vi "Change File True.vi"(0 "error in":errorcluster, 1 "Numeric in":u16, 2 "Ring":refnum<vi>) -> (7 "error out":errorcluster, 8 "Numeric out":u16, 9 "Change song?":bool)   [LabVIEW 2019]
doc: "Checks if the Ring has been changed or if the application has finished reading the audio file and sends a boolean value depending the condition was true."
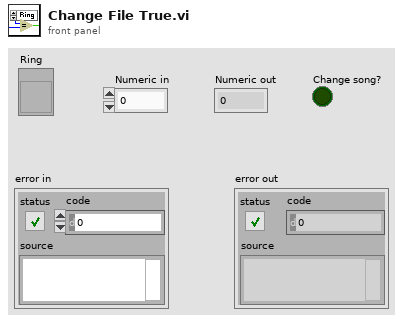
[diagram p1: front panel]
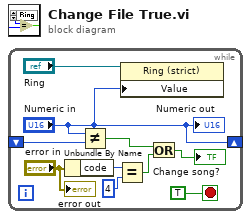
[diagram p0: block diagram]
diagram:
  n1 = while {
    shift-right: ["Numeric in"] -> _
    shift-left: _ -> [w9]
    stop <- TRUE stop-if-true
    n2 = Unbundle By Name("error in") -> ("code"=w7:i32)
    n3 = Not Equal?(x="Numeric in", y=w9) -> (x != y?=w4:bool)
    n4 = Equal?(x=w7, y=4) -> (x = y?=w6:bool)
    n5 = property class="Ring (strict)"(reference="Ring", "Value"="Numeric in") -> ()  [unwired: 1 in, 2 out]
    n6 = Or(x=w4, y=w6) -> (x .or. y?=→"Change song?":bool)
    "Numeric out" <- "Numeric in"
    "error out" <- "error in"
  }
